vi "Mapcluster.vi"() -> ()   [LabVIEW 2009]
uses:
  <vilib>/Analysis/Matrix/Datatypes/RealMatrix.ctl
  <vilib>/Analysis/Matrix/NI_Matrix.lvlib
panel:
  out "time":u32
  out "Coordinates":cluster{"X":dbl, "Y":dbl}[](array[cluster])=[{"X"=1.0, "Y"=24.0}, {"X"=4.0, "Y"=11.0}, {"X"=6.0, "Y"=9.0}, {"X"=6.0, "Y"=3.0}, {"X"=14.0, "Y"=9.0}, {"X"=14.0, "Y"=11.0}, {"X"=14.0, "Y"=13.0}, {"X"=10.0, "Y"=15.0}, {"X"=10.0, "Y"=17.0}, {"X"=20.0, "Y"=17.0}, {"X"=21.0, "Y"=14.0}, {"X"=21.0, "Y"=5.0}, {"X"=23.0, "Y"=1.0}]
  out "Path":i32[](array[numeric])=[12]
  out "Map":T1=[[0.0, 0.0, 0.0, 0.0, 0.0, 0.0, 0.0, 0.0, 0.0, 0.0, 0.0, 0.0, 0.0, 0.0, 0.0, 0.0, 0.0, 0.0, 0.0, 0.0, 0.0, 0.0, 0.0, 0.0, 0.0], [0.0, 0.0, 0.0, 0.0, 0.0, 0.0, 0.0, 0.0, 0.0, 0.0, 0.0, 0.0, 0.0, 0.0, 0.0, 0.0, 0.0, 0.0, 0.0, 0.0, 0.0, 0.0, 0.0, 2.0, 0.0], [0.0, 0.0, 0.0, 0.0, 0.0, 0.0, 0.0, 0.0, 0.0, 0.0, 0.0, 0.0, 0.0, 0.0, 0.0, 0.0, 0.0, 0.0, 0.0, 0.0, 0.0, 0.0, 0.0, 0.0, 0.0], [0.0, 0.0, 0.0, 0.0, 0.0, 0.0, 0.0, 0.0, 0.0, 0.0, 0.0, 0.0, 0.0, 0.0, 0.0, 0.0, 0.0, 0.0, 0.0, 0.0, 0.0, 0.0, 0.0, 0.0, 0.0], [0.0, 0.0, 0.0, 0.0, 0.0, 0.0, 0.0, 0.0, 0.0, 0.0, 0.0, 2.0, 0.0, 0.0, 0.0, 0.0, 0.0, 0.0, 0.0, 0.0, 0.0, 0.0, 0.0, 0.0, 0.0], [0.0, 0.0, 0.0, 0.0, 0.0, 0.0, 0.0, 0.0, 0.0, 0.0, 0.0, 0.0, 1.0, 1.0, 1.0, 1.0, 1.0, 1.0, 1.0, 1.0, 1.0, 1.0, 1.0, 1.0, 1.0], [0.0, 0.0, 0.0, 2.0, 0.0, 0.0, 0.0, 0.0, 0.0, 2.0, 0.0, 0.0, 1.0, 1.0, 1.0, 1.0, 1.0, 1.0, 1.0, 1.0, 1.0, 1.0, 1.0, 1.0, 1.0], [0.0, 0.0, 0.0, 0.0, 1.0, 1.0, 1.0, 1.0, 1.0, 0.0, 0.0, 0.0, 1.0, 1.0, 1.0, 1.0, 1.0, 1.0, 1.0, 1.0, 1.0, 1.0, 1.0, 1.0, 1.0], [0.0, 0.0, 0.0, 0.0, 1.0, 1.0, 1.0, 1.0, 1.0, 0.0, 0.0, 0.0, 1.0, 0.0, 0.0, 0.0, 0.0, 0.0, 0.0, 0.0, 0.0, 0.0, 0.0, 0.0, 0.0], [0.0, 0.0, 0.0, 0.0, 1.0, 1.0, 1.0, 1.0, 1.0, 0.0, 0.0, 0.0, 1.0, 0.0, 0.0, 0.0, 0.0, 0.0, 0.0, 0.0, 0.0, 0.0, 0.0, 0.0, 0.0], [1.0, 1.0, 1.0, 1.0, 1.0, 1.0, 1.0, 1.0, 1.0, 0.0, 0.0, 0.0, 1.0, 0.0, 0.0, 2.0, 0.0, 2.0, 0.0, 0.0, 0.0, 0.0, 0.0, 0.0, 0.0], [1.0, 1.0, 1.0, 1.0, 1.0, 1.0, 1.0, 1.0, 1.0, 0.0, 0.0, 0.0, 1.0, 0.0, 0.0, 0.0, 1.0, 0.0, 0.0, 0.0, 0.0, 0.0, 0.0, 0.0, 0.0], [1.0, 1.0, 1.0, 1.0, 1.0, 1.0, 1.0, 1.0, 1.0, 0.0, 0.0, 0.0, 1.0, 0.0, 0.0, 0.0, 1.0, 0.0, 0.0, 0.0, 0.0, 0.0, 0.0, 0.0, 0.0], [1.0, 1.0, 1.0, 1.0, 1.0, 1.0, 1.0, 1.0, 1.0, 0.0, 0.0, 0.0, 1.0, 0.0, 0.0, 0.0, 1.0, 0.0, 0.0, 0.0, 0.0, 0.0, 0.0, 0.0, 0.0], [0.0, 0.0, 0.0, 0.0, 0.0, 0.0, 0.0, 0.0, 0.0, 2.0, 0.0, 2.0, 0.0, 2.0, 0.0, 0.0, 1.0, 0.0, 0.0, 0.0, 0.0, 0.0, 0.0, 0.0, 0.0], [0.0, 0.0, 0.0, 0.0, 0.0, 0.0, 0.0, 0.0, 0.0, 0.0, 0.0, 0.0, 0.0, 0.0, 0.0, 0.0, 1.0, 0.0, 0.0, 0.0, 0.0, 0.0, 0.0, 0.0, 0.0], [1.0, 1.0, 1.0, 1.0, 1.0, 1.0, 1.0, 1.0, 1.0, 1.0, 1.0, 1.0, 1.0, 1.0, 1.0, 1.0, 1.0, 0.0, 0.0, 0.0, 0.0, 0.0, 0.0, 0.0, 0.0], [1.0, 1.0, 1.0, 1.0, 1.0, 1.0, 1.0, 1.0, 1.0, 1.0, 1.0, 1.0, 1.0, 1.0, 1.0, 1.0, 1.0, 0.0, 0.0, 0.0, 0.0, 0.0, 0.0, 0.0, 0.0], [1.0, 1.0, 1.0, 1.0, 1.0, 1.0, 1.0, 1.0, 1.0, 1.0, 1.0, 1.0, 1.0, 1.0, 1.0, 1.0, 1.0, 0.0, 0.0, 0.0, 0.0, 0.0, 0.0, 0.0, 0.0], [1.0, 1.0, 1.0, 1.0, 1.0, 1.0, 1.0, 1.0, 1.0, 1.0, 1.0, 1.0, 1.0, 1.0, 1.0, 1.0, 1.0, 0.0, 0.0, 0.0, 0.0, 0.0, 0.0, 0.0, 0.0], [0.0, 0.0, 0.0, 0.0, 0.0, 0.0, 0.0, 0.0, 0.0, 0.0, 0.0, 0.0, 0.0, 0.0, 0.0, 0.0, 0.0, 2.0, 0.0, 0.0, 0.0, 0.0, 0.0, 0.0, 0.0], [0.0, 0.0, 0.0, 0.0, 0.0, 2.0, 0.0, 0.0, 0.0, 0.0, 0.0, 0.0, 0.0, 0.0, 2.0, 0.0, 0.0, 0.0, 0.0, 0.0, 0.0, 0.0, 0.0, 0.0, 0.0], [0.0, 0.0, 0.0, 0.0, 0.0, 0.0, 1.0, 1.0, 1.0, 1.0, 1.0, 1.0, 1.0, 1.0, 0.0, 0.0, 0.0, 0.0, 0.0, 0.0, 0.0, 0.0, 0.0, 0.0, 0.0], [0.0, 0.0, 0.0, 0.0, 0.0, 0.0, 1.0, 1.0, 1.0, 1.0, 1.0, 1.0, 1.0, 1.0, 0.0, 0.0, 0.0, 0.0, 0.0, 0.0, 0.0, 0.0, 0.0, 0.0, 0.0], [0.0, 2.0, 0.0, 0.0, 0.0, 0.0, 1.0, 1.0, 1.0, 1.0, 1.0, 1.0, 1.0, 1.0, 0.0, 0.0, 0.0, 0.0, 0.0, 0.0, 0.0, 0.0, 0.0, 0.0, 0.0]]
  in  "Corners 2":cluster{"X":i32, "Y":i32}[](array[cluster])=[{"X"=4, "Y"=11}, {"X"=6, "Y"=9}, {"X"=6, "Y"=3}, {"X"=14, "Y"=9}, {"X"=14, "Y"=11}, {"X"=14, "Y"=13}, {"X"=10, "Y"=15}, {"X"=10, "Y"=17}, {"X"=20, "Y"=17}, {"X"=21, "Y"=14}, {"X"=21, "Y"=5}]
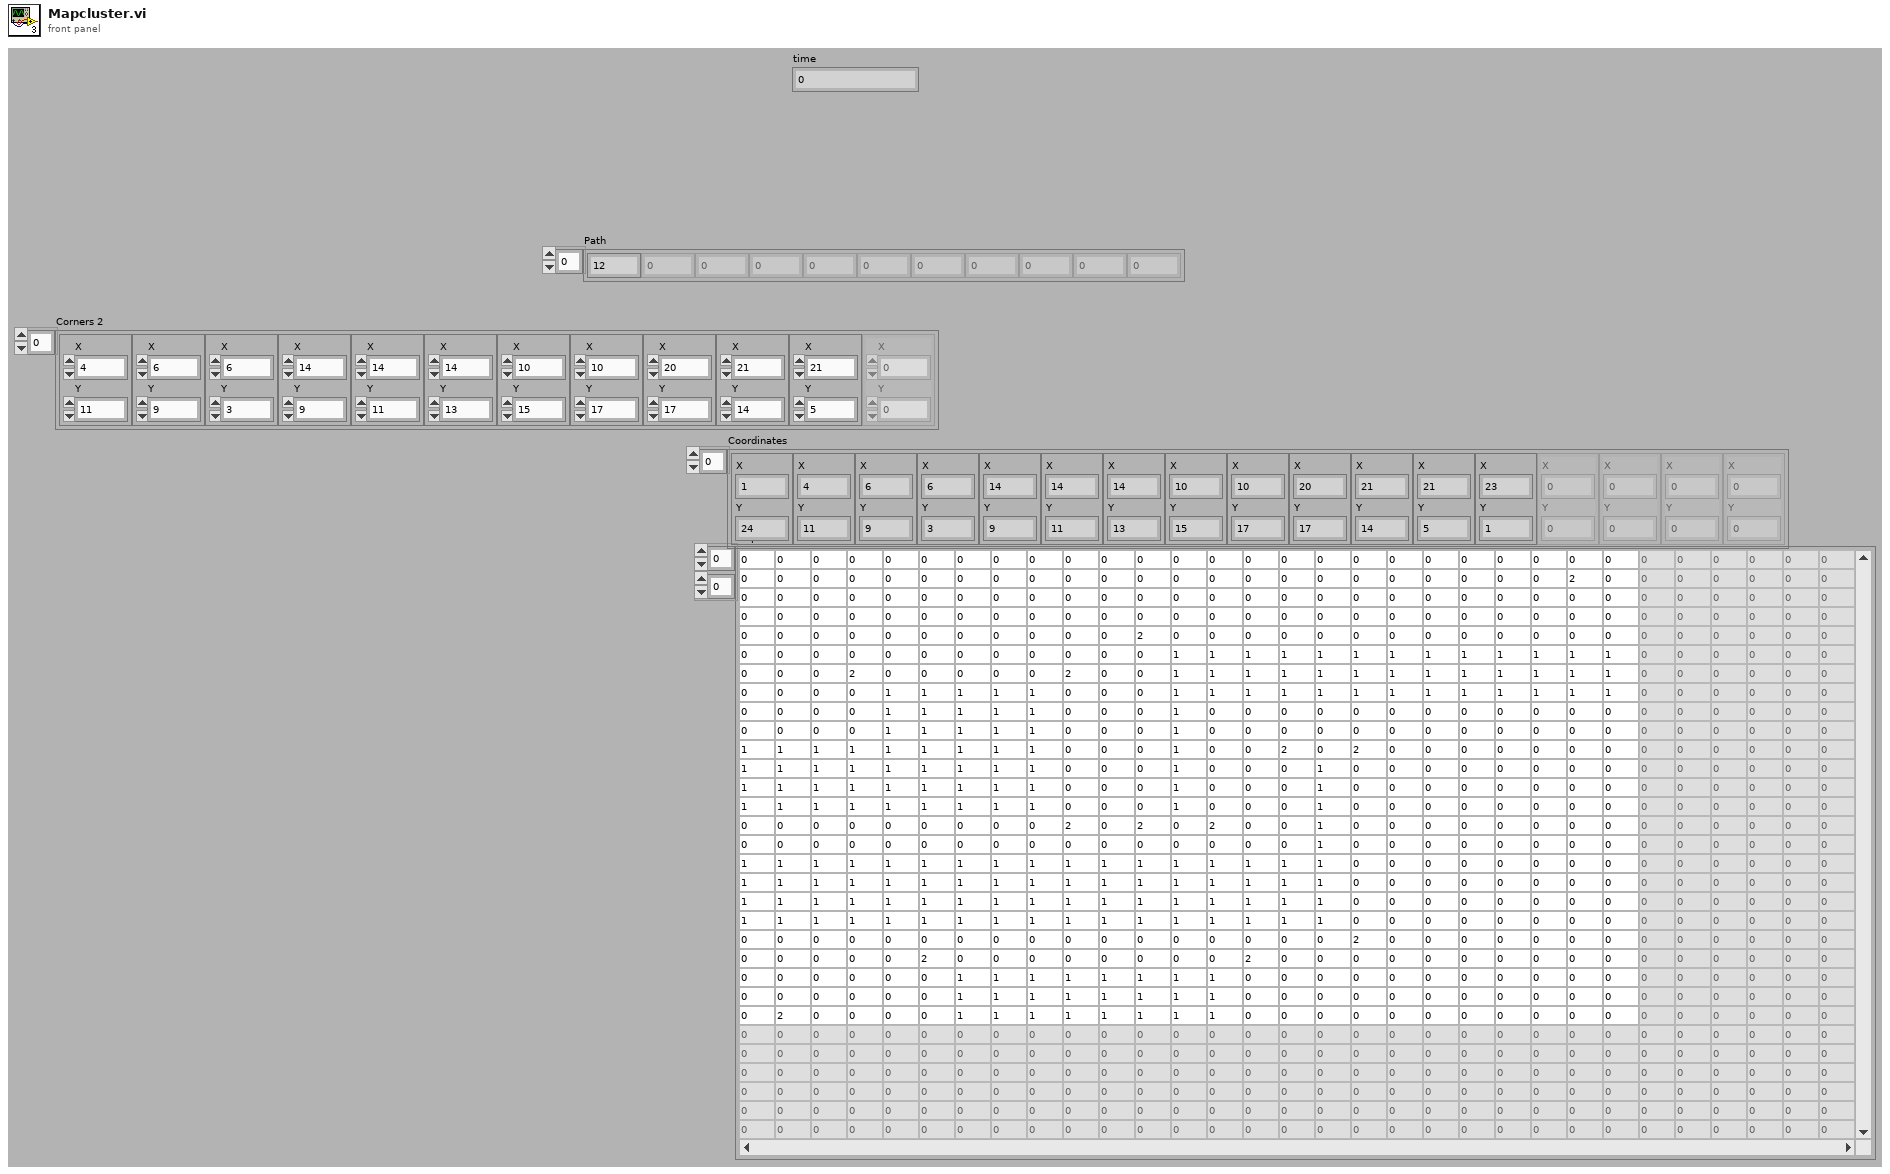
[diagram p1: front panel]
types:
  T1 = typedef "NI_Matrix.lvlib/RealMatrix.ctl" = dbl[][]
  T2 = cluster{"Robot":cluster{"X":i32, "Y":i32, "Bearing":i32}, "Map":i8[][], "Goal":cluster{"X":i32, "Y":i32}, "Corners":cluster{"X":i32, "Y":i32}[]}
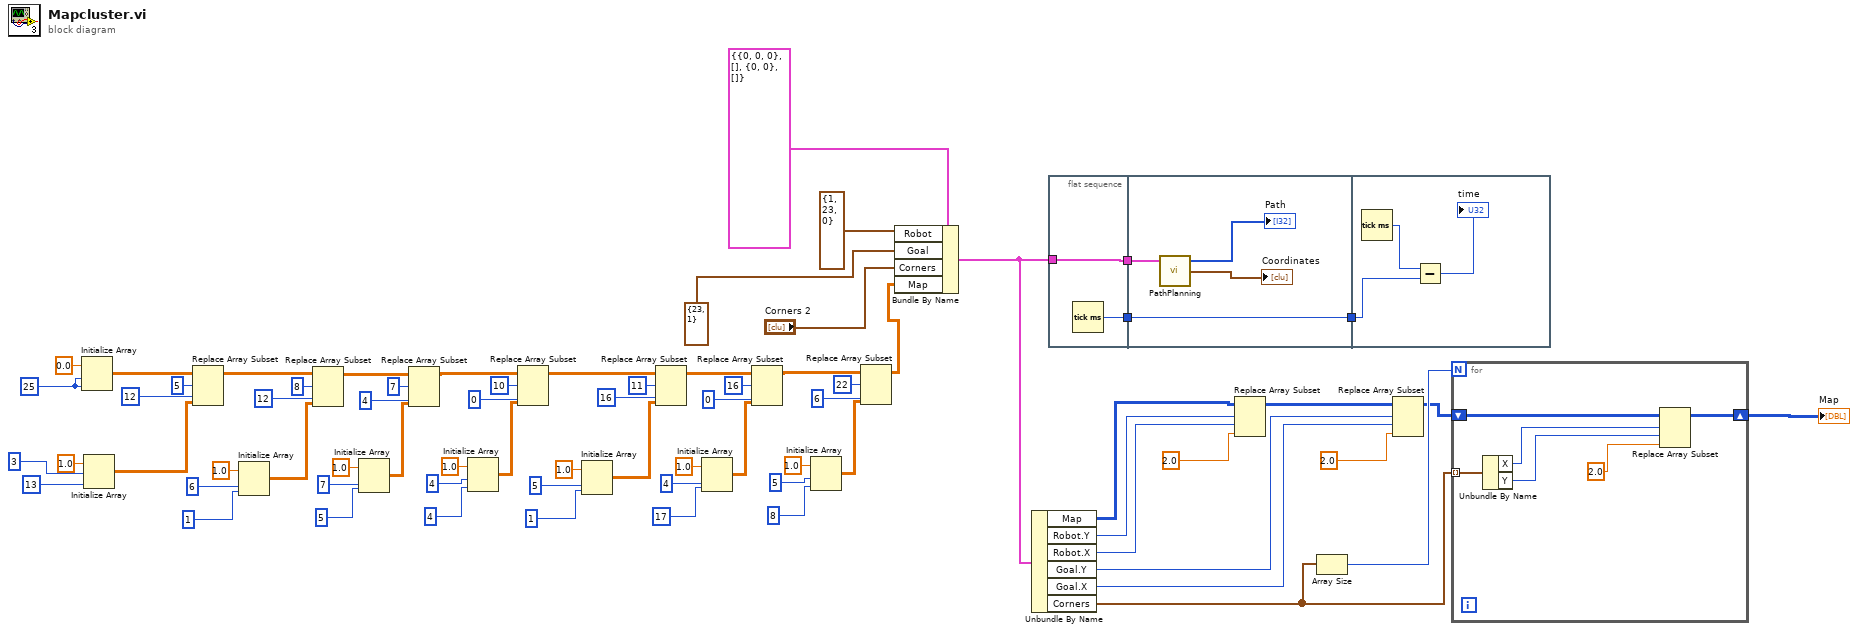
[diagram p0: block diagram]
diagram:
  w67 = 25 ("dimension size")
  n1 = Initialize Array(0.0 ("element"), w67, w67) -> (w6:dbl[][])
  n2 = Initialize Array(1.0 ("element"), 3 ("dimension size"), 13 ("dimension size")) -> (w64:dbl[][])
  n3 = Replace Array Subset(array=w6, new element=w64, index (row)=5, index (col)=12 ("disabled index (col)")) -> (w61:dbl[][])
  n4 = Initialize Array(1.0 ("element"), 6 ("dimension size"), 1 ("dimension size")) -> (w58:dbl[][])
  n5 = Replace Array Subset(array=w61, new element=w58, index (row)=8, index (col)=12 ("disabled index (col)")) -> (w54:dbl[][])
  n6 = Initialize Array(1.0 ("element"), 7 ("dimension size"), 5 ("dimension size")) -> (w50:dbl[][])
  n7 = Replace Array Subset(array=w54, new element=w50, index (row)=7, index (col)=4 ("disabled index (col)")) -> (w31:dbl[][])
  n8 = Initialize Array(1.0 ("element"), 4 ("dimension size"), 4 ("dimension size")) -> (w32:dbl[][])
  n9 = Replace Array Subset(array=w31, new element=w32, index (row)=10, index (col)=0 ("disabled index (col)")) -> (w8:dbl[][])
  n10 = Initialize Array(1.0 ("element"), 5 ("dimension size"), 1 ("dimension size")) -> (w25:dbl[][])
  n11 = Replace Array Subset(array=w8, new element=w25, index (row)=11, index (col)=16 ("disabled index (col)")) -> (w22:dbl[][])
  n12 = Initialize Array(1.0 ("element"), 4 ("dimension size"), 17 ("dimension size")) -> (w18:dbl[][])
  n13 = Replace Array Subset(array=w22, new element=w18, index (row)=16, index (col)=0 ("disabled index (col)")) -> (w11:dbl[][])
  n14 = Initialize Array(1.0 ("element"), 5 ("dimension size"), 8 ("dimension size")) -> (w12:dbl[][])
  n15 = Replace Array Subset(array=w11, new element=w12, index (row)=22, index (col)=6 ("disabled index (col)")) -> (w5:dbl[][])
  n16 = Bundle By Name(cluster=T2 {"Robot"={"X"=0, "Y"=0, "Bearing"=0}, "Map"=[], "Goal"={"X"=0, "Y"=0}, "Corners"=[]} ("Map 2"), "Robot"=cluster{i32, i32, i32} {1, 23, 0}, "Goal"=cluster{"X":i32, "Y":i32} {"X"=23, "Y"=1}, "Corners"="Corners 2", "Map"=w5) -> (w4:T2)
  n17 = Unbundle By Name(w4) -> ("Map"=w47:i8[][], "Robot.Y"=w46:i32, "Robot.X"=w45:i32, "Goal.Y"=w43:i32, "Goal.X"=w42:i32, "Corners"=w40:cluster{"X":i32, "Y":i32}[])
  n18 = flat-sequence {
    tunnel: w4 -> [w74]
    tunnel: [w74] -> w3
    tunnel: [w73] -> w1
    tunnel: w3 -> [w76]
    tunnel: [w75] -> w2
    tunnel: w1 -> [w75]
    tunnel: w2 -> [w79]
    frame #0 {
      n19 = Tick Count (ms)() -> (millisecond timer value=w73:u32)
    }
    frame #1 {
      n20 = call "PathPlanning.vi"("Map & Nodes"=w76) -> ("Path"=→"Path":i32[], "Coordinates"=→"Coordinates":cluster{"X":dbl, "Y":dbl}[])  [unwired: 1 in, 1 out]
    }
    frame #2 {
      n21 = Tick Count (ms)() -> (millisecond timer value=w80:u32)
      n22 = Subtract(x=w80, y=w79) -> (x-y=→"time":u32)
    }
  }
  n23 = Replace Array Subset(array=w47, new element=2.0 ("element"), index (row)=w46, index (col)=w45) -> (w44:i8[][])
  n24 = Array Size(array=w40) -> (size(s)=w41:i32)
  n25 = Replace Array Subset(array=w44, new element=2.0 ("element"), index (row)=w43, index (col)=w42) -> (w39:i8[][])
  n26 = for {
    N: w41 -> [_]
    tunnel: w40 -> [w87] mode=indexing
    shift-right: [w83] -> w38
    shift-left: w39 -> [w86]
    n27 = Unbundle By Name(w87) -> ("X"=w85:i32, "Y"=w84:i32)
    n28 = Replace Array Subset(array=w86, new element=2.0 ("element"), index (row)=w85, index (col)=w84) -> (w83:i8[][])
  }
  "Map" <- w38
